vi "Configure SWR Timer Times.vi"(8 "error in (no error)":errorcluster, 9 "skip time, s":u8, 10 "count time, s":u8, 11 "HFP Gen in":refnum<class "PL HFP Generator.lvclass">) -> (0 "error out":errorcluster, 3 "HFP Gen out":refnum<class "PL HFP Generator.lvclass">)   [LabVIEW 2015, in "PL HFP Generator.lvclass"]
doc: "Configures SWR timer count and skip times. RF is blocked if Pref exceeds threshold for a specified count time. If Pref is below threshold for a specified skip time, timer is reset."
uses:
  PL HFP Generator.lvclass
  <vilib>/plasmapper/PL Modbus Client/PL Modbus Client.lvclass
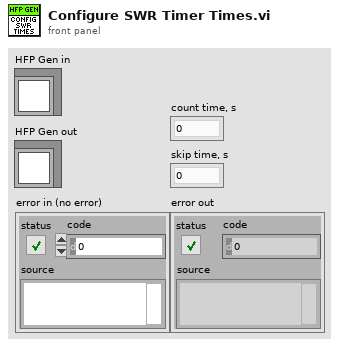
[diagram p1: front panel]
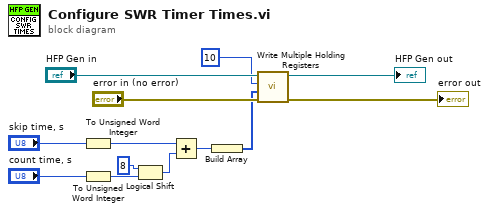
[diagram p0: block diagram]
diagram:
  n1 = To Unsigned Word Integer(number="skip time, s") -> (unsigned 16bit integer=w4:u16)
  n2 = To Unsigned Word Integer(number="count time, s") -> (unsigned 16bit integer=w7:u16)
  n3 = Logical Shift(y=i16 8, x=w7) -> (x << y=w3:u16)
  n4 = Add(x=w4, y=w3) -> (x+y=w5:u16)
  n5 = Build Array(w5) -> (w8:u16[])
  n6 = call <vilib>:"Write Multiple Holding Registers.vi"("error in (no error)"="error in (no error)", "values"=w8, "address"=u16 10, "MODBUS in"="HFP Gen in") -> ("error out"=→"error out":errorcluster, "MODBUS out"=→"HFP Gen out":refnum<class "PL HFP Generator.lvclass">)  [unwired: 6 in]
